vi "SVFA Zoom Power Spectrum.vi"   [LabVIEW 2017]
doc: "Computes the zoom power spectrum of <B>scaled signal [EU]</B> and <B>zoom settings</B>. Data accumulates each time this VI is called. However, it returns a new spectrum only when sufficient data accumulates. Indicators and subsequent processing should only be called when <B>new spectrum available</B> is TRUE. Wire data to the <B>scaled signal [EU]</B> input to determine the polymorphic instance to use or manually select the instance."
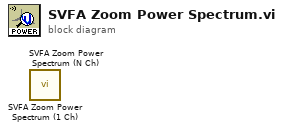
[diagram p0: block diagram]
diagram:
  n1 = call <vilib>:"SVFA Zoom Power Spectrum (1 Ch).vi"() -> ()  [unwired: 13 in, 7 out]
  n2 = call <vilib>:"SVFA Zoom Power Spectrum (N Ch).vi"() -> ()  [unwired: 13 in, 7 out]
